vi "Sensor_m.vi"() -> ()   [LabVIEW 2018]
panel:
  out "Sensor_{m}":dbl[](array[numeric]) format="%.1f"
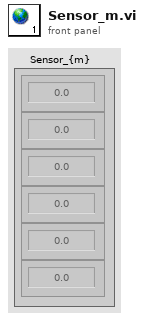
[diagram p1: front panel]
diagram:
